vi "Initialize.vi"() -> (0 "error out":errorcluster, 3 ".NET Refnum out":refnum<k24>)   [LabVIEW 2019, in "ESP301.lvlib"]
uses:
  ESP301.lvlib
  Newport.ESP301.CommandInterface
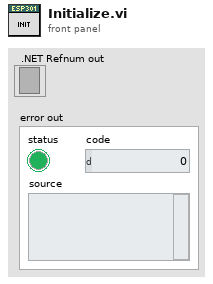
[diagram p1: front panel]
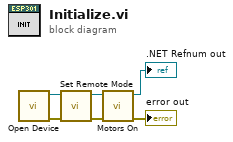
[diagram p0: block diagram]
diagram:
  n1 = call "Open Device.vi"() -> ("error out"=w6:errorcluster, ".NET Refnum out"=w5:refnum<k24>)  [unwired: 10 in]
  n2 = call "Set Remote Mode.vi"("error in (no error)"=w6, ".NET Refnum in"=w5) -> ("error out"=w3:errorcluster, ".NET Refnum out"=w4:refnum<k24>)  [unwired: 8 in]
  n3 = call "Motors On.vi"("error in (no error)"=w3, ".NET Refnum in"=w4) -> ("error out"=→"error out":errorcluster, ".NET Refnum out"=→".NET Refnum out":refnum<k24>)  [unwired: 8 in]
